vi "Counter_ReadPulseWidth.vi"(3 "Task ID":u32) -> (1 "pulse width":cluster{"high period":dbl, "low period":dbl})   [LabVIEW 2015]
uses:
  Windows/System32/AdvLvDaq.dll
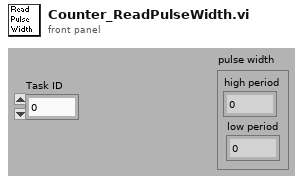
[diagram p1: front panel]
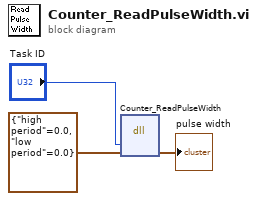
[diagram p0: block diagram]
diagram:
  n1 = dll-call lib="C:/Windows/System32/AdvLvDaq.dll" fn="Counter_ReadPulseWidth"("taskId"="Task ID", "arg2"=cluster{"high period":dbl, "low period":dbl} {"high period"=0.0, "low period"=0.0}) -> ("arg2"=→"pulse width":cluster{"high period":dbl, "low period":dbl})  [unwired: 4 in, 3 out]
